vi "Table_AssertAllItems_Tests.vi"(8 "error in":errorcluster) -> (0 "error out":errorcluster)   [LabVIEW 2016, in "DronaTest.lvlib"]
uses:
  DronaTest.lvlib
  APIs/Stimulus/ControlValue/SetValueAuto.vi
  APIs/Assert/AssertControlValue/Controls/Table/AssertAllItems.vi
  <vilib>/addons/_JKI Toolkits/Caraya/classes/Assert/Assert Equal Value_Variant.vi
  <vilib>/addons/_JKI Toolkits/Caraya/classes/Test/Test.lvclass
  <vilib>/SLL Toolkit/SLL Debug/SLL Debug.lvlib
  Drona.lvlib
  <vilib>/addons/_JKI Toolkits/Caraya/classes/Assert/Assert.lvclass
  APIs/Get/GetControlRef/GetControlRef.lvlib
  APIs/Stimulus/ControlValue/ControlValue.lvlib
  APIs/Assert/AssertControlValue/Controls/Table/AssertTable.lvlib
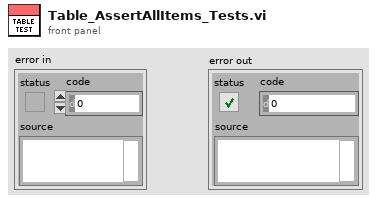
[diagram p1: front panel]
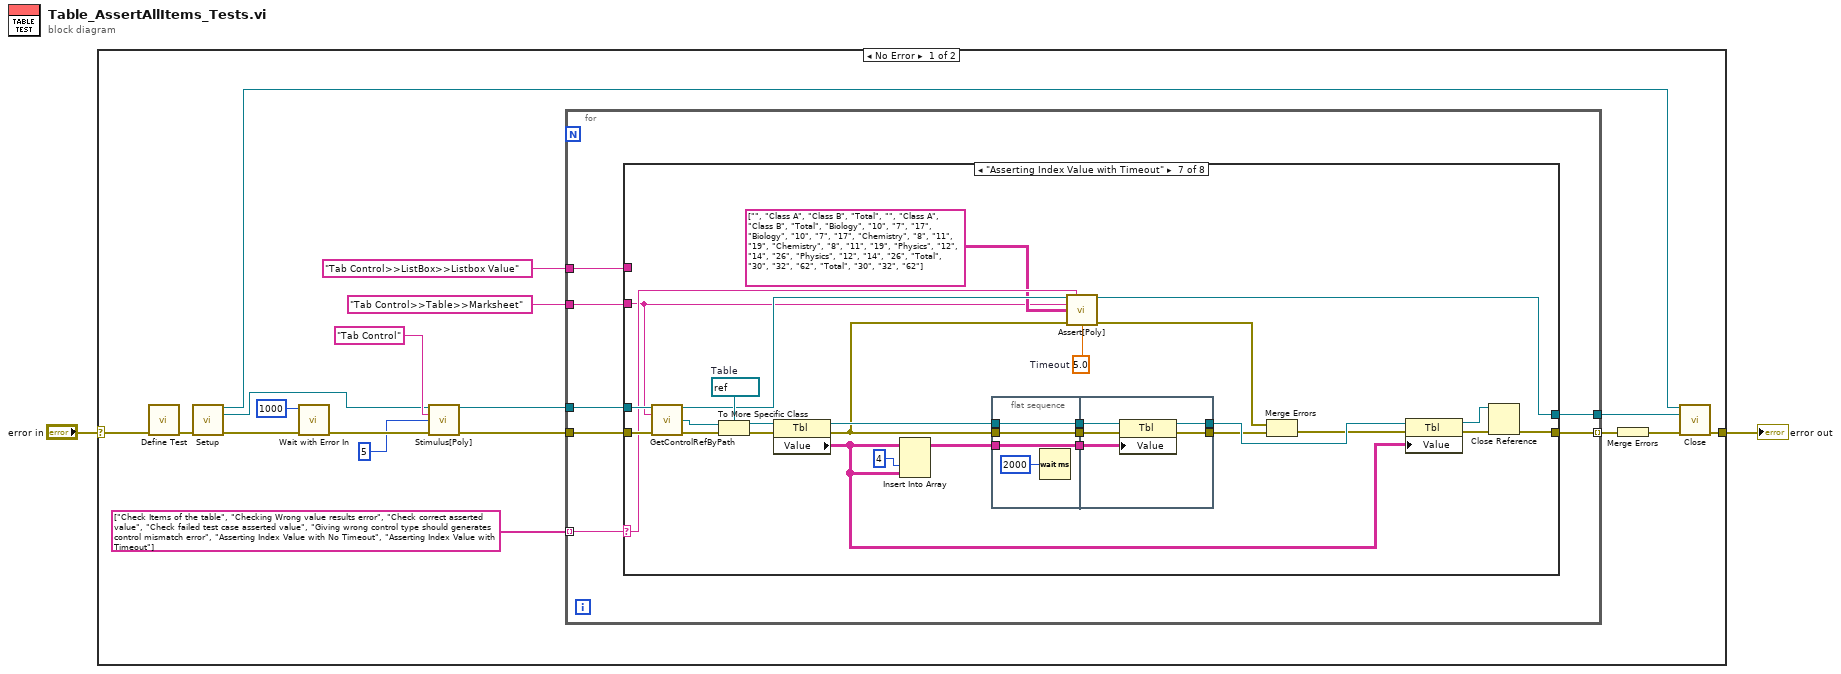
[diagram p0: block diagram]
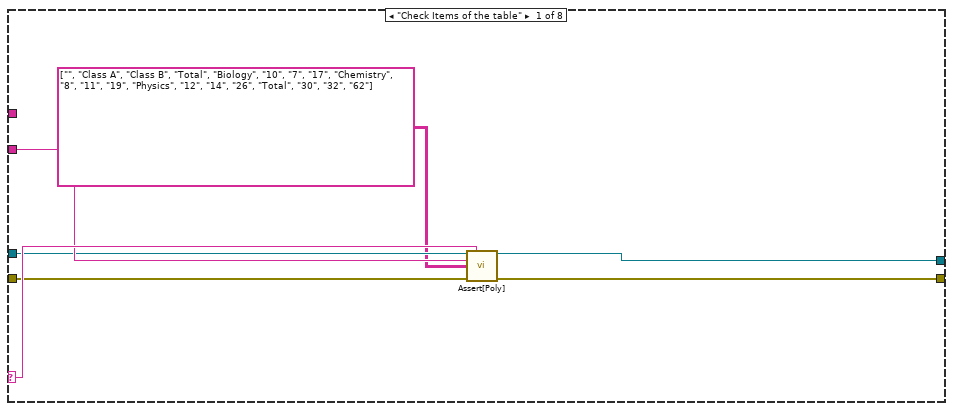
[diagram p2: hidden frame]
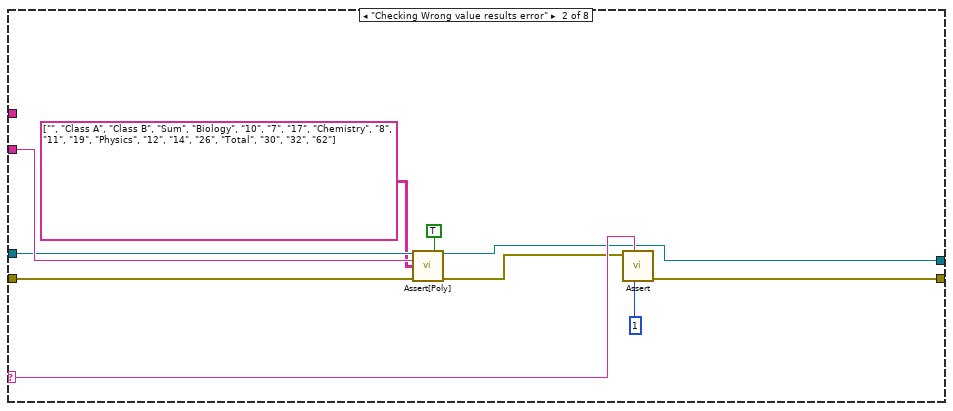
[diagram p3: hidden frame]
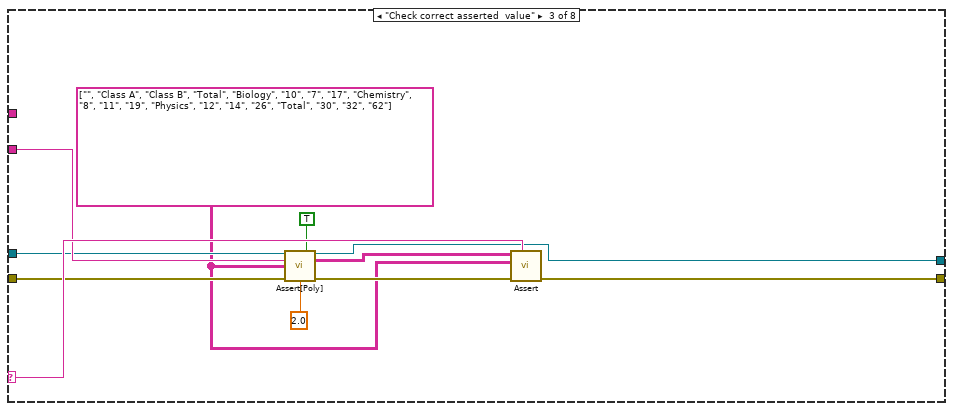
[diagram p4: hidden frame]
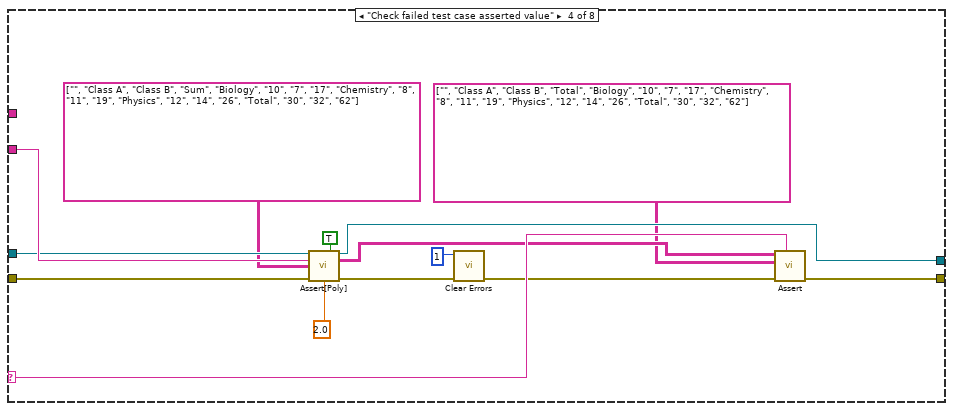
[diagram p5: hidden frame]
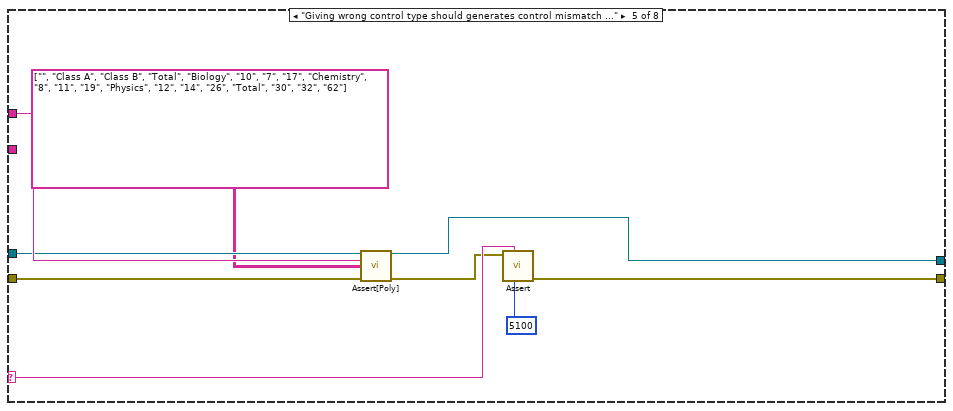
[diagram p6: hidden frame]
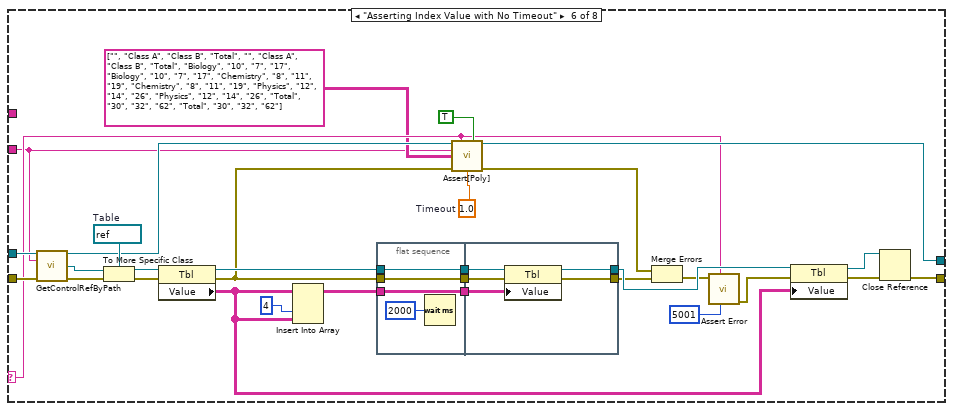
[diagram p7: hidden frame]
diagram:
  n1 = case shown="No Error" "error in" {
    selector: "error in" -> [w20 w158]
    tunnel: [w3 w158] -> w1
    frame No Error {
      n2 = call <vilib>:"Define Test.vi"("error in (no error)"=w20) -> ("error out"=w9:errorcluster)  [unwired: 9 in, 1 out]
      n3 = call "Setup.vi"("error in"=w9) -> ("Application Ref"=w5:refnum<vi>, "VI Reference Out"=w7:refnum<vi>, "error out"=w8:errorcluster)  [unwired: 12 in]
      n4 = call <vilib>:"Wait with Error In.vi"("error in (no error)"=w8, "milliseconds to wait"=u32 1000) -> ("error out"=w18:errorcluster)  [unwired: 9 in]
      n5 = call-poly "Stimulus[Poly].vi"("VI Reference In"=w7, "Control Path"="Tab Control", "Value (Signaling)"=5, "error in"=w18) -> ("VI Reference Out"=w14:refnum<vi>, "error out"=w17:errorcluster)  [unwired: 10 in]
      n6 = for {
        tunnel: w14 -> [w23]
        tunnel: "Tab Control>>Table>>Marksheet" ("Control Path") -> [w21]
        tunnel: "Tab Control>>ListBox>>Listbox Value" ("Control Path") -> [w22]
        tunnel: string[] ["Check Items of the table", "Checking Wrong value results error", "Check correct asserted  value", "Check failed test case asserted value", "Giving wrong control type should generates control mismatch error", "Asserting Index Value with No Timeout", "Asserting Index Value with Timeout"] -> [w27] mode=indexing
        tunnel: [w25] -> w4
        tunnel: w17 -> [w24]
        tunnel: [w26] -> w10 mode=indexing
        n7 = case shown="\"Asserting Index Value with Timeout\"" w27 {
          selector: w27 -> [w32 w43 w54 w68 w77 w84 w136 _]
          tunnel: w24 -> [w30 w37 w50 w64 w72 w109 w146 w157]
          tunnel: w23 -> [w29 w36 w49 w63 w71 w107 w144 w156]
          tunnel: w21 -> [w31 w41 w53 w67 _ w79 w119 _]
          tunnel: w22 -> [_ _ _ _ w74 _ _ _]
          tunnel: [w34 w44 w55 w69 w78 w96 w132 w157] -> w26
          tunnel: [w33 w40 w52 w66 w73 w100 w137 w156] -> w25
          frame "Check Items of the table" {
            n8 = call-poly "Assert[Poly].vi"("VI Reference In"=w29, "Test Label"=w32, "Control Path"=w31, "Item Value"=string[][] [["", "Class A", "Class B", "Total"], ["Biology", "10", "7", "17"], ["Chemistry", "8", "11", "19"], ["Physics", "12", "14", "26"], ["Total", "30", "32", "62"]] ("Marksheet"), "Error In"=w30) -> ("VI Reference Out"=w33:refnum<vi>, "Error Out"=w34:errorcluster)  [unwired: 8 in, 1 out]
          }
          frame "Checking Wrong value results error" {
            n9 = call-poly "Assert[Poly].vi"("VI Reference In"=w36, "Assert Only? (F)"=TRUE, "Control Path"=w41, "Item Value"=string[][] [["", "Class A", "Class B", "Sum"], ["Biology", "10", "7", "17"], ["Chemistry", "8", "11", "19"], ["Physics", "12", "14", "26"], ["Total", "30", "32", "62"]] ("Marksheet"), "Error In"=w37) -> ("VI Reference Out"=w40:refnum<vi>, "Error Out"=w39:errorcluster)  [unwired: 8 in, 1 out]
            n10 = call-poly <vilib>:"Assert.vi"("error code (1)"=1, "Label"=w43, "Error?"=w39) -> ("error out"=w44:errorcluster)  [unwired: 7 in, 1 out]
          }
          frame "Check correct asserted  value" {
            w45 = string[][] [["", "Class A", "Class B", "Total"], ["Biology", "10", "7", "17"], ["Chemistry", "8", "11", "19"], ["Physics", "12", "14", "26"], ["Total", "30", "32", "62"]] ("Marksheet")
            n11 = call-poly "Assert[Poly].vi"("VI Reference In"=w49, "Assert Only? (F)"=TRUE, "Control Path"=w53, "Item Value"=w45, "Error In"=w50, "Timeout(5 sec)"=2.0) -> ("VI Reference Out"=w52:refnum<vi>, "Asserted Value"=w47:string[][], "Error Out"=w48:errorcluster)  [unwired: 7 in]
            n12 = call-poly <vilib>:"Assert.vi"("Label"=w54, "error in (no error)"=w48, "Y"=w45, "X"=w47) -> ("error out"=w55:errorcluster)  [unwired: 6 in, 1 out]
          }
          frame "Check failed test case asserted value" {
            n13 = call-poly "Assert[Poly].vi"("VI Reference In"=w63, "Assert Only? (F)"=TRUE, "Control Path"=w67, "Item Value"=string[][] [["", "Class A", "Class B", "Sum"], ["Biology", "10", "7", "17"], ["Chemistry", "8", "11", "19"], ["Physics", "12", "14", "26"], ["Total", "30", "32", "62"]] ("Marksheet"), "Error In"=w64, "Timeout(5 sec)"=2.0) -> ("VI Reference Out"=w66:refnum<vi>, "Asserted Value"=w61:string[][], "Error Out"=w62:errorcluster)  [unwired: 7 in]
            n14 = call <vilib>:"Clear Errors.vi"("error in (no error)"=w62, "specific error code to clear (0: all)"=1) -> ("error out"=w60:errorcluster)  [unwired: 4 in, 1 out]
            n15 = call-poly <vilib>:"Assert.vi"("Label"=w68, "error in (no error)"=w60, "Y"=string[][] [["", "Class A", "Class B", "Total"], ["Biology", "10", "7", "17"], ["Chemistry", "8", "11", "19"], ["Physics", "12", "14", "26"], ["Total", "30", "32", "62"]] ("Marksheet"), "X"=w61) -> ("error out"=w69:errorcluster)  [unwired: 6 in, 1 out]
          }
          frame "Giving wrong control type should generates control mismatch error" {
            n16 = call-poly "Assert[Poly].vi"("VI Reference In"=w71, "Control Path"=w74, "Item Value"=string[][] [["", "Class A", "Class B", "Total"], ["Biology", "10", "7", "17"], ["Chemistry", "8", "11", "19"], ["Physics", "12", "14", "26"], ["Total", "30", "32", "62"]] ("Marksheet"), "Error In"=w72) -> ("VI Reference Out"=w73:refnum<vi>, "Error Out"=w75:errorcluster)  [unwired: 9 in, 1 out]
            n17 = call-poly <vilib>:"Assert.vi"("error code (1)"=5100, "Label"=w77, "Error?"=w75) -> ("error out"=w78:errorcluster)  [unwired: 7 in, 1 out]
          }
          frame "Asserting Index Value with No Timeout" {
            w93 = 1.0  # Timeout
            w104 = refnum<vi> refnum  # Table
            n18 = call "GetControlRefByPath.vi"("VI Reference In"=w107, "Control Path"=w79, "error In"=w109) -> ("VI Reference Out"=w101:refnum<vi>, "Ctl Refnum"=w105:refnum<vi>, "error out"=w108:errorcluster)  [unwired: 10 in]
            n19 = To More Specific Class(target class=w104, reference=w105, error in=w108) -> (specific class reference=w103:refnum<vi>, error out=w106:errorcluster)
            n20 = property on="Property Node" class="Tbl"(reference=w103, error in=w106) -> (reference out=w99:refnum<vi>, error out=w92:errorcluster, "Value"=w81:string[][])
            n21 = Insert Into Array(array=w81, index (col)=4 ("disabled index (col)"), new element=w81) -> (w102:string[][])  [unwired: 1 in]
            n22 = flat-sequence {
              tunnel: w92 -> [w111]
              tunnel: w99 -> [w112]
              tunnel: w102 -> [w113]
              tunnel: [w113] -> w90
              tunnel: [w112] -> w89
              tunnel: [w111] -> w88
              tunnel: [w116] -> w95
              tunnel: [w114] -> w91
              tunnel: w90 -> [w118]
              tunnel: w89 -> [w117]
              tunnel: w88 -> [w115]
              frame #0 {
                n23 = Wait (ms)(milliseconds to wait=u32 2000) -> ()  [unwired: 1 out]
              }
              frame #1 {
                n24 = property on="Property Node" class="Tbl"(reference=w117, error in=w115, "Value"=w118) -> (reference out=w116:refnum<vi>, error out=w114:errorcluster)
              }
            }
            n25 = call-poly "Assert[Poly].vi"("VI Reference In"=w101, "Test Label"=w84, "Assert Only? (F)"=TRUE, "Control Path"=w79, "Item Value"=string[][] [["", "Class A", "Class B", "Total", "", "Class A", "Class B", "Total"], ["Biology", "10", "7", "17", "Biology", "10", "7", "17"], ["Chemistry", "8", "11", "19", "Chemistry", "8", "11", "19"], ["Physics", "12", "14", "26", "Physics", "12", "14", "26"], ["Total", "30", "32", "62", "Total", "30", "32", "62"]] ("Value"), "Error In"=w92, "Timeout(5 sec)"=w93) -> ("VI Reference Out"=w100:refnum<vi>, "Error Out"=w98:errorcluster)  [unwired: 6 in, 1 out]
            n26 = Merge Errors(w98, w91) -> (w87:errorcluster)
            n27 = call <vilib>:"Assert Error.vi"("error code (1)"=5001, "Label"=w84, "Error?"=w87) -> ("error out"=w86:errorcluster)  [unwired: 7 in, 1 out]
            n28 = property on="Property Node" class="Tbl"(reference=w95, error in=w86, "Value"=w81) -> (reference out=w94:refnum<vi>, error out=w97:errorcluster)
            n29 = Close Reference(reference=w94, error in (no error)=w97) -> (error out=w96:errorcluster)
          }
          frame "Asserting Index Value with Timeout" {
            w123 = 5.0  # Timeout
            w141 = refnum<vi> refnum  # Table
            n30 = call "GetControlRefByPath.vi"("VI Reference In"=w144, "Control Path"=w119, "error In"=w146) -> ("VI Reference Out"=w138:refnum<vi>, "Ctl Refnum"=w142:refnum<vi>, "error out"=w145:errorcluster)  [unwired: 10 in]
            n31 = To More Specific Class(target class=w141, reference=w142, error in=w145) -> (specific class reference=w140:refnum<vi>, error out=w143:errorcluster)
            n32 = property on="Property Node" class="Tbl"(reference=w140, error in=w143) -> (reference out=w135:refnum<vi>, error out=w129:errorcluster, "Value"=w122:string[][])
            n33 = Insert Into Array(array=w122, index (col)=4 ("disabled index (col)"), new element=w122) -> (w139:string[][])  [unwired: 1 in]
            n34 = flat-sequence {
              tunnel: w129 -> [w148]
              tunnel: w135 -> [w149]
              tunnel: w139 -> [w150]
              tunnel: [w150] -> w126
              tunnel: [w149] -> w125
              tunnel: [w148] -> w124
              tunnel: [w153] -> w131
              tunnel: [w151] -> w127
              tunnel: w126 -> [w155]
              tunnel: w125 -> [w154]
              tunnel: w124 -> [w152]
              frame #0 {
                n35 = Wait (ms)(milliseconds to wait=u32 2000) -> ()  [unwired: 1 out]
              }
              frame #1 {
                n36 = property on="Property Node" class="Tbl"(reference=w154, error in=w152, "Value"=w155) -> (reference out=w153:refnum<vi>, error out=w151:errorcluster)
              }
            }
            n37 = call-poly "Assert[Poly].vi"("VI Reference In"=w138, "Test Label"=w136, "Control Path"=w119, "Item Value"=string[][] [["", "Class A", "Class B", "Total", "", "Class A", "Class B", "Total"], ["Biology", "10", "7", "17", "Biology", "10", "7", "17"], ["Chemistry", "8", "11", "19", "Chemistry", "8", "11", "19"], ["Physics", "12", "14", "26", "Physics", "12", "14", "26"], ["Total", "30", "32", "62", "Total", "30", "32", "62"]] ("Value"), "Error In"=w129, "Timeout(5 sec)"=w123) -> ("VI Reference Out"=w137:refnum<vi>, "Error Out"=w134:errorcluster)  [unwired: 7 in, 1 out]
            n38 = Merge Errors(w134, w127) -> (w128:errorcluster)
            n39 = property on="Property Node" class="Tbl"(reference=w131, error in=w128, "Value"=w122) -> (reference out=w130:refnum<vi>, error out=w133:errorcluster)
            n40 = Close Reference(reference=w130, error in (no error)=w133) -> (error out=w132:errorcluster)
          }
          frame Default {
          }
        }
      }
      n41 = Merge Errors(w10) -> (w6:errorcluster)
      n42 = call "Close.vi"("Application Ref"=w5, "VI Reference"=w4, "error in"=w6) -> ("error out"=w3:errorcluster)  [unwired: 12 in]
    }
    frame Error {
    }
  }
  "error out" <- w1
